vi "Create System.vi"(8 "error in (no error)":errorcluster, 10 "System Name":string, 11 "VolatusConfig in":refnum<class "VolatusConfig.lvclass">) -> (0 "error out":errorcluster, 2 "System":refnum<class "System Config.lvclass">, 3 "VolatusConfig out":refnum<class "VolatusConfig.lvclass">)   [LabVIEW 2020, in "VolatusConfig.lvlib" / "VolatusConfig.lvclass"]
uses:
  VolatusConfig.lvclass
  System/System Config.lvclass
  Meta Type.ctl
  VolatusConfig.lvclass/VolatusConfig.ctl
  lv-cdm/CDM-Config/Config Lookup/Match Meta.vi
  lv-cdm/CDM-Config/Config Element/Owner.vi
  lv-cdm/CDM-Config/Config Manager/Lookup Descendant.vi
  lv-cdm/CDM-Config/Config Filter/Config Lookup.lvclass
  VolatusConfig.lvlib
  lv-cdm/CDM-Config/Config Element/Config Element.lvclass
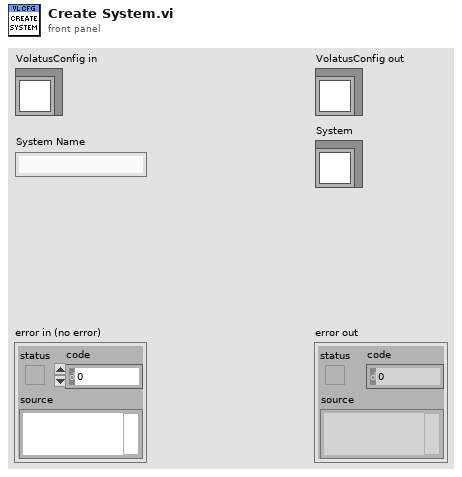
[diagram p1: front panel]
types:
  T1 = typedef "VolatusConfig.lvlib/Meta Type.ctl" = enum16{"UNKNOWN", "VL_System", "VL_Cluster", "VL_Node", "VL_Task", "VL_Group", "VL_Channel", "VL_Task_List", "VL_Scaling", "VL_Sensor", "VL_Sensor_List", "VL_Scale"}
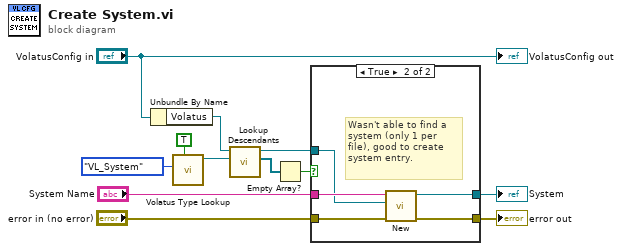
[diagram p0: block diagram]
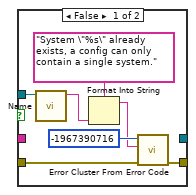
[diagram p2: hidden frame]
diagram:
  n1 = Unbundle By Name("VolatusConfig in") -> ("Volatus"=w10:refnum<class "Config Element.lvclass">)
  n2 = call "Volatus Type Lookup.vi"("Don't Recurse Past Match (F)"=TRUE, "Meta Type"=Meta_Type."VL_System") -> ("Config Lookup out"=w3:refnum<class "Config Lookup.lvclass">)  [unwired: 8 in, 1 out]
  n3 = call "Lookup Descendants.vi"("Lookup"=w3, "Config Element in"=w10) -> ("Descendants"=w2:refnum<class "Config Element.lvclass">[], "Config Element out"=w4:refnum<class "Config Element.lvclass">)  [unwired: 7 in, 1 out]
  n4 = Empty Array?(array=w2) -> (empty?=w1:bool)
  n5 = case shown="True" w1 {
    tunnel: "System Name" -> [_ w24]
    tunnel: [_ w23] -> w9
    tunnel: [w18 w22] -> w8
    tunnel: "error in (no error)" -> [w19 w21]
    tunnel: w4 -> [w14 w20]
    frame False {
      n6 = call "Name.vi"("Config Element in"=w14) -> ("Name"=w13:string)  [unwired: 9 in, 1 out]
      n7 = Format Into String(format string="System \"%s\" already exists, a config can only contain a single system.", w13) -> (resulting string=w16:string)  [unwired: 2 in, 1 out]
      n8 = call <vilib>:"Error Cluster From Error Code.vi"("error in (no error)"=w19, "error message (\"\")"=w16, "error code (0)"=-1967390716) -> ("error out"=w18:errorcluster)  [unwired: 6 in]
    }
    frame True {
      # "Wasn't able to find a system (only 1 per file), good to create system entry."
      n9 = call "New.vi"("error in (no error)"=w21, "Parent"=w20, "System Name"=w24) -> ("error out"=w22:errorcluster, "System out"=w23:refnum<class "System Config.lvclass">)  [unwired: 6 in, 1 out]
    }
  }
  "error out" <- w8
  "System" <- w9
  "VolatusConfig out" <- "VolatusConfig in"
